vi "write16bitTiff-Bigtiff.vi"(2 "16-bit pixmap x, y":u16[][](array[numeric]), 3 "Text":string, 4 "file path":path=path "\\\\till-server\\work/Software_IT/Labview/Colibri/Library/tiff/examples/test-16bit-write-Bigtiff.tif") -> (0 "error out":errorcluster)   [LabVIEW 2011]
panel:
  in  "BigTiff,Endian":u16(ring)=257 items=["Big-Endian"=0, "Native"=1, "Little-Endian"=2, "BigTiff-Big-Endian"=256, "Bigtiff,Native"=257, "Biftiff,Littleendian"=258]
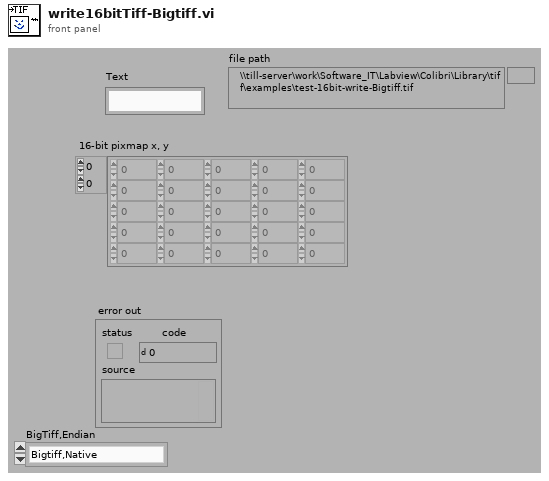
[diagram p1: front panel]
types:
  T1 = cluster{"Tiff refnum":refnum<file>, "BigTiff,Endian":u16}
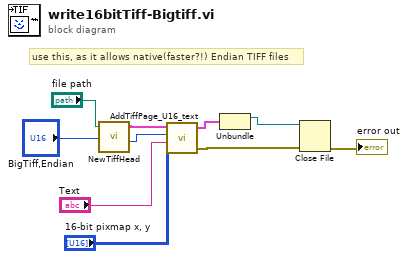
[diagram p0: block diagram]
diagram:
  # "use this, as it allows native(faster?!) Endian TIFF files"
  n1 = call "NewTiffHead.vi"("file path"="file path", "BigTiff,Endian"="BigTiff,Endian") -> ("TIFF file"=w6:T1, "Place for first IFD (8,eof-position)"=w1:u64)  [unwired: 2 in, 1 out]
  n2 = call "AddTiffPage_U16_text.vi"("TIFF file"=w6, "After last DIROffset"=w1, "Text"="Text", "16-bit pixmap x, y"="16-bit pixmap x, y") -> ("TIFF file"=w5:T1, "error out"=w2:errorcluster)  [unwired: 1 in, 1 out]
  n3 = Unbundle(w5) -> ("Tiff refnum"=w9:refnum<file>)  [unwired: 1 out]
  n4 = Close File(refnum=w9, error in=w2) -> (error out=→"error out":errorcluster)  [unwired: 1 out]
